vi "Wind Farm #1 Cluster.vi"() -> (0 "Cluster":T1)   [LabVIEW 2009]
doc: "This is the cluster for Wind Farm #1.\n\nAAL 9/09"
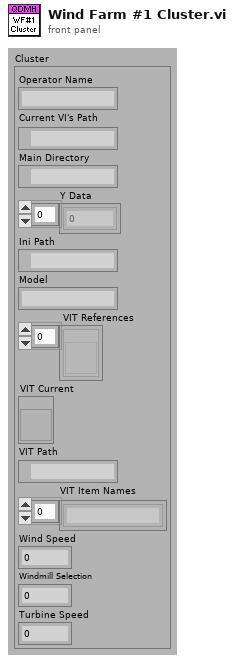
[diagram p1: front panel]
types:
  T1 = cluster{"Operator Name":string, "Current VI's Path":path, "Main Directory":path, "Y Data":dbl[], "Ini Path":path, "Model":string, " VIT References":refnum<vi>[], "VIT Current":refnum<vi>, "VIT Path":path, "VIT Item Names ":string[], "Wind Speed":dbl, "Windmill Selection":i32, "Turbine Speed":dbl}
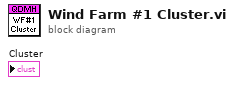
[diagram p0: block diagram]
diagram:
